vi "multiple inverters.vi"() -> ()   [LabVIEW 2018]
uses:
  <vilib>/Plasmionique/MB Master/MB_Master_TCP/MB_Master_TCP.lvclass
  <vilib>/Plasmionique/MB Master/MB Master.lvlib
  93058b94-2cfa-412c-aaea-c37432080e69.vi
  52964f07-62a9-4f69-bcdd-33621c3da344.vi
  12cb2fec-a066-4508-9dd1-fd50a70bf569.vi
  6f8febb2-9bf6-4d29-9751-6b01666fea3d.vi
  b6474e31-9fa1-4c1d-99b5-b6bb53db0f46.vi
  f1a4f3b6-1467-4be9-9e5d-893fa62d5f27.vi
  d295411a-7b3b-4ec3-9029-25cb82dd415e.vi
  31b17e4d-b534-4e5a-9b0d-c0ca24deb87e.vi
  b632eabe-c25f-4dbe-95ee-deebe4b0f4b1.vi
  7138b5ac-df4f-457e-8d99-eea4f057fb14.vi
  7631bdb0-5171-4193-ab14-fa7f9aada4b6.vi
  93641b55-29e7-4da1-9539-9e254f8d73b5.vi
  C:/Program Files (x86)/National Instruments/LabVIEW 2018/vi.lib/Plasmionique/MB Master/MB_Master/MB_Master.lvclass
panel:
  out "Curtailment  Complete":bool
  out "Power Factor Complete":bool
  out "Set Up Complete":bool
  in  "1200 Inverter IP":string
  in  "1086 Inverter IP":string
  in  "1084 Inverter IP":string
  in  "Setup Curtailment and Power Factor":bool
  in  "Send Curtailment":bool
  in  "Send Power Factor":bool
  out "Setup Runtime (s)":u16
  out "Curtailment Runtime (s)":dbl
  out "Power Factor Runtime (s)":dbl
  in  "stop":bool
  in  "Curtailment % (28-100)":enum16{""}(ring)
  in  "power Factor Setpoint":enum16{""}(ring)
  in  "Inverter Select":T1(ring)
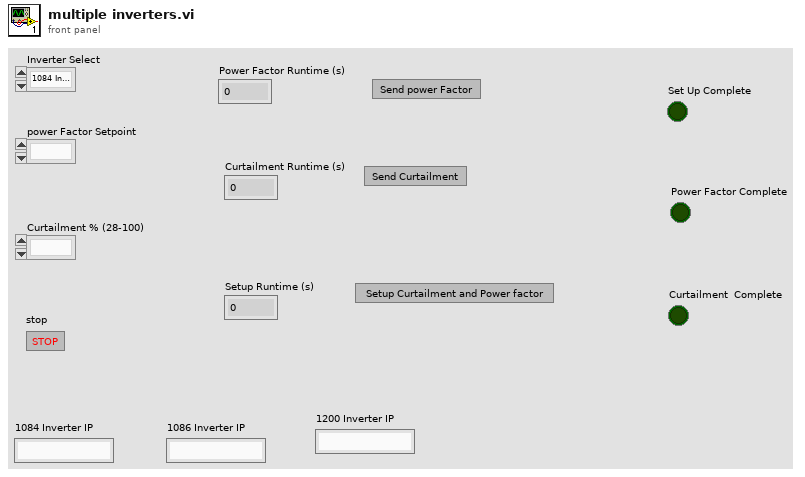
[diagram p1: front panel]
types:
  T1 = enum16{"1084 Inverter", "1086 Inverter ", "1200 Inverter"}
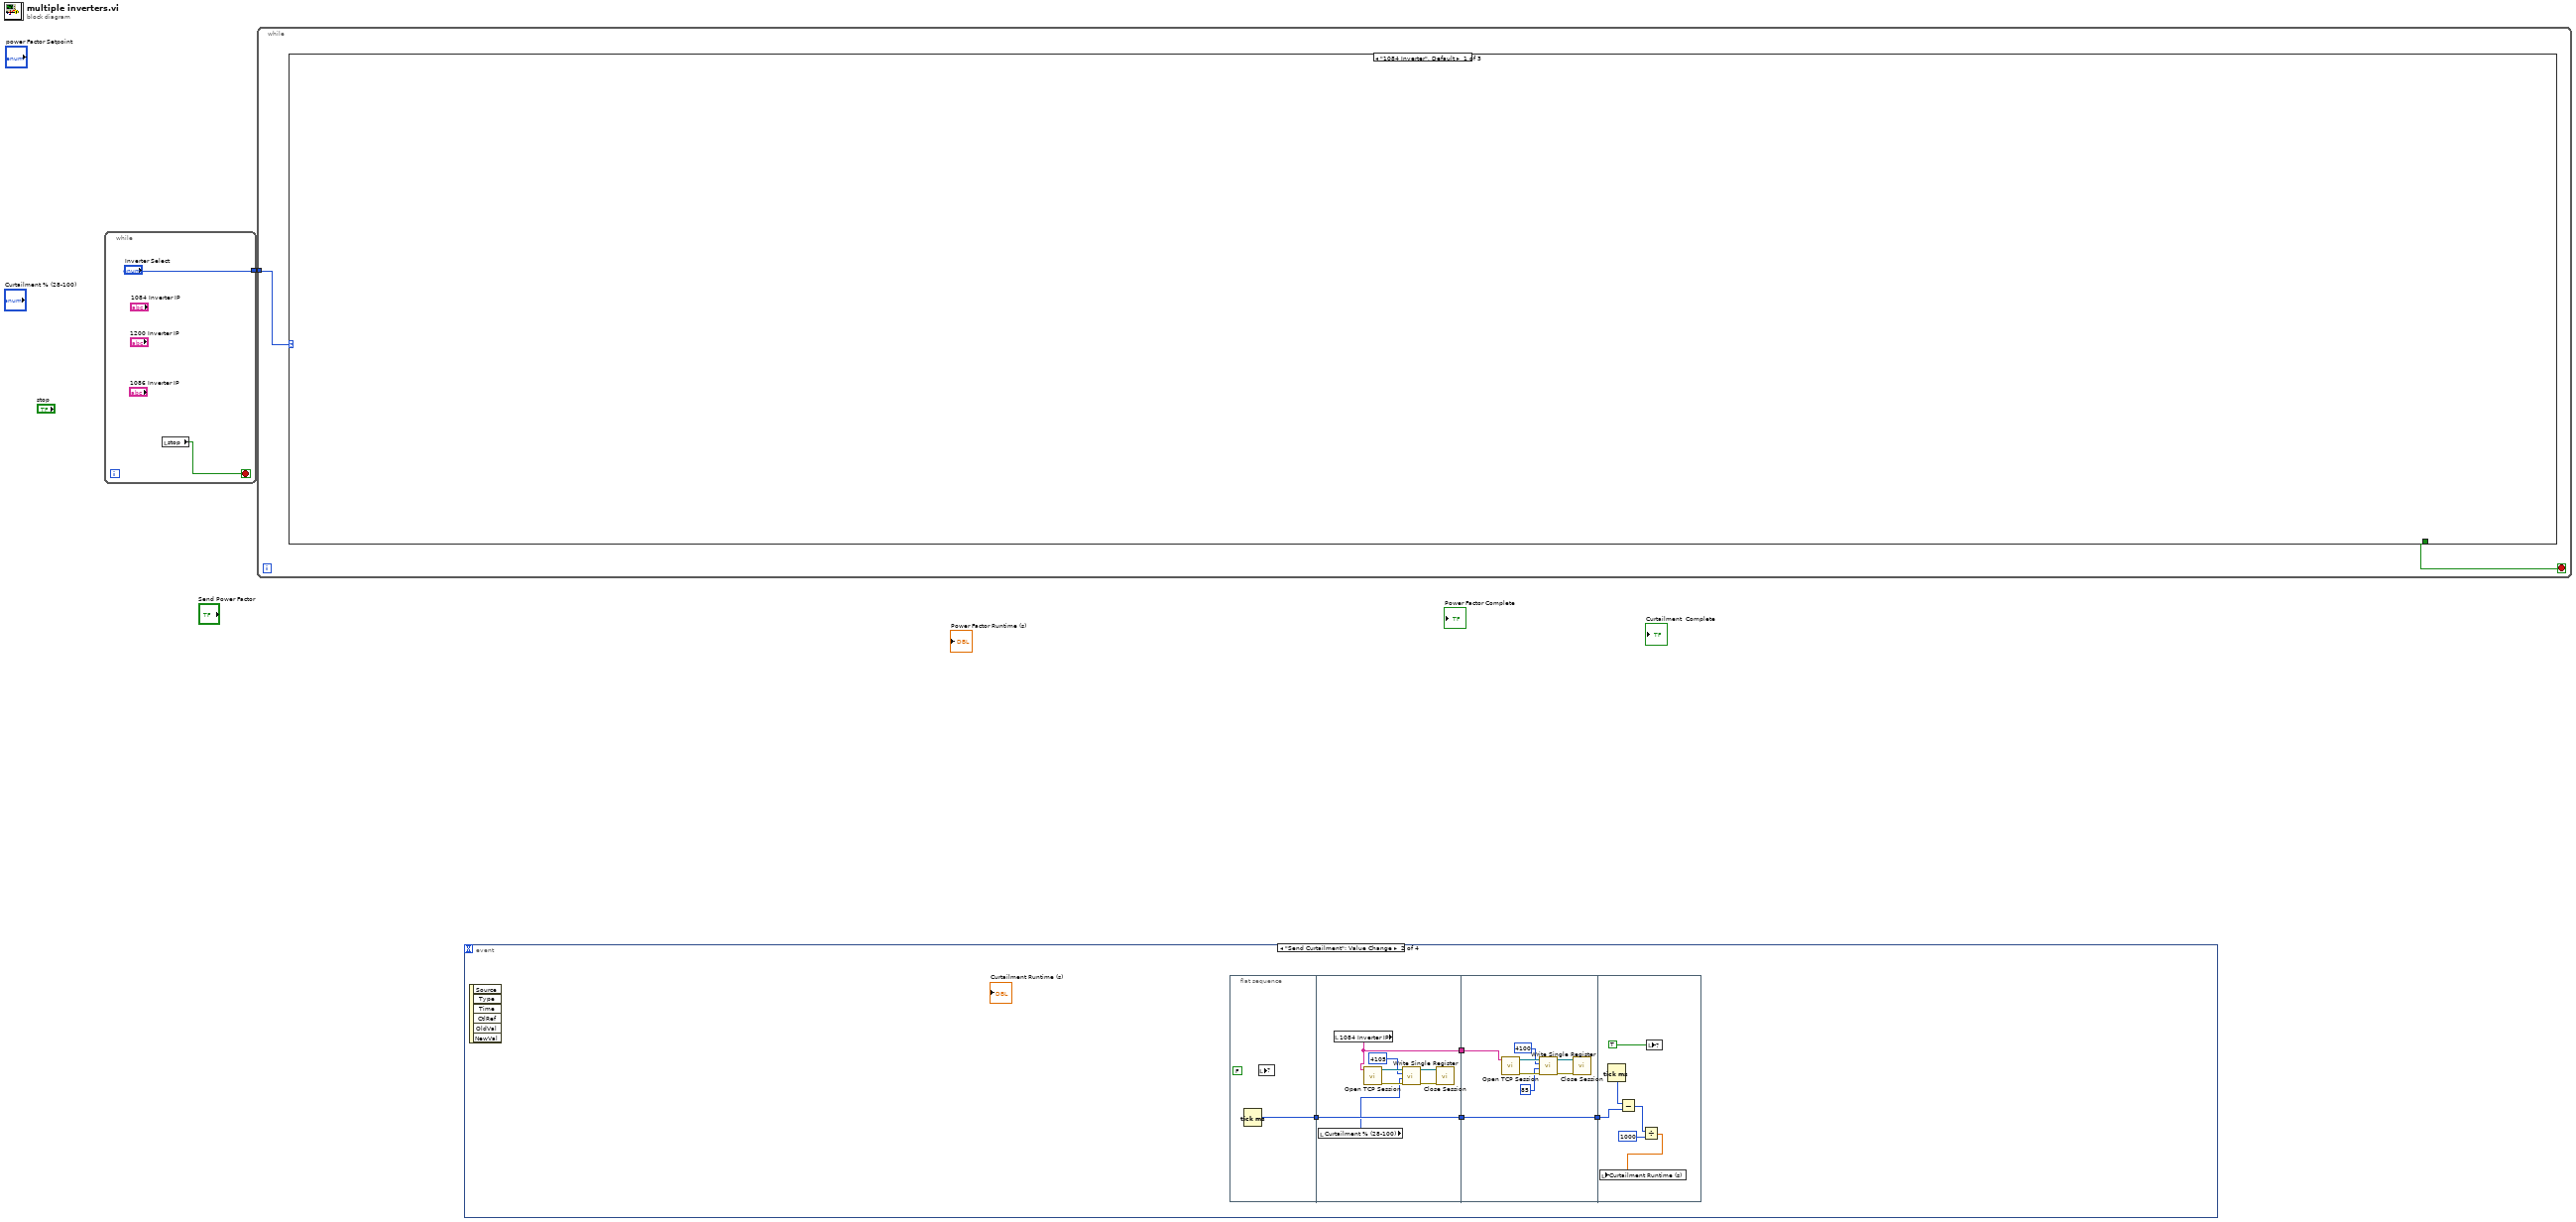
[diagram p0: block diagram]
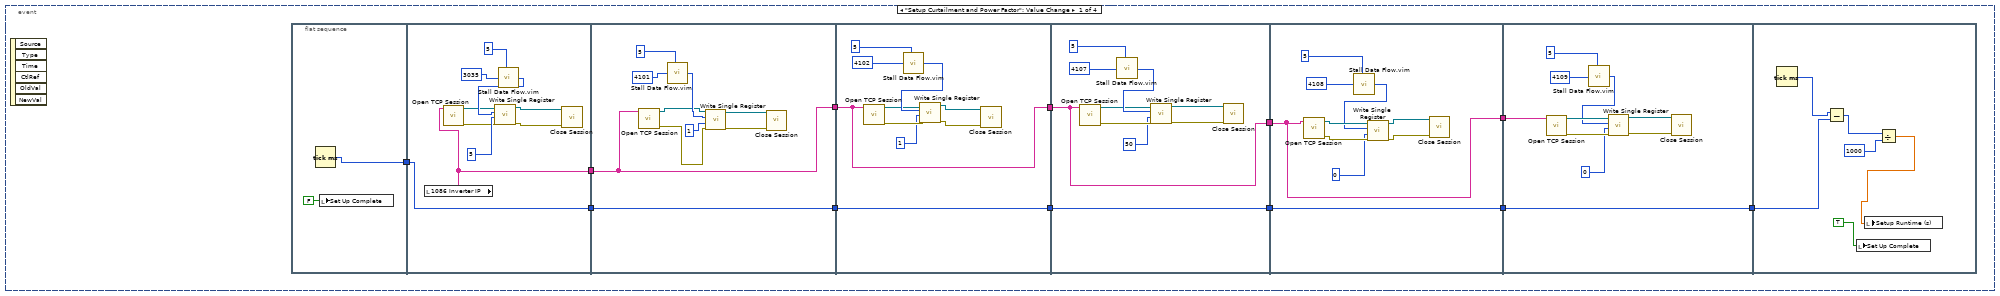
[diagram p2: hidden frame]
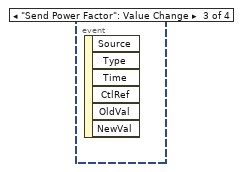
[diagram p3: hidden frame]
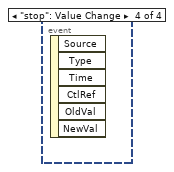
[diagram p4: hidden frame]
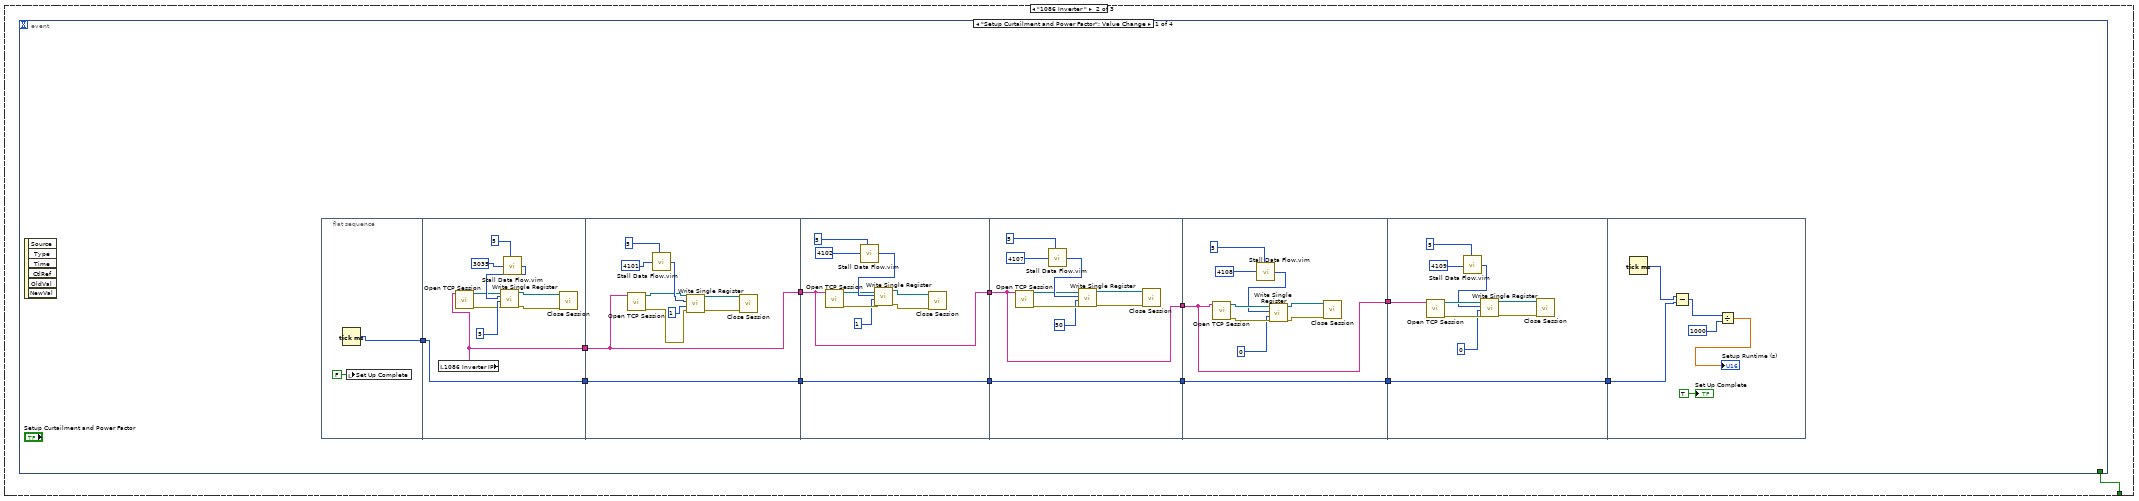
[diagram p5: hidden frame]
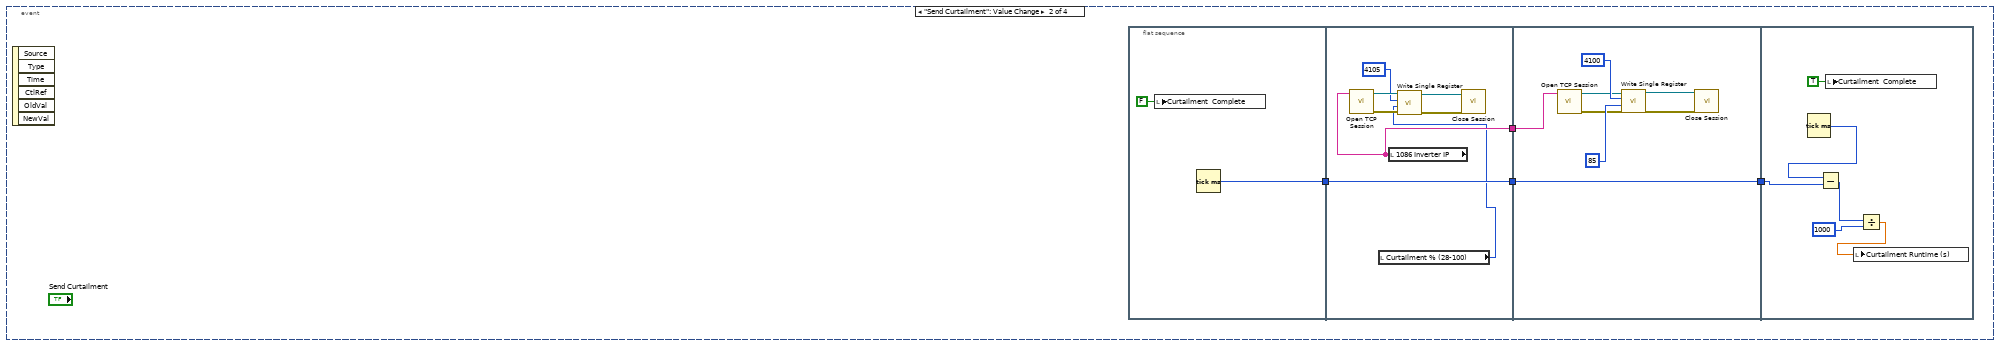
[diagram p6: hidden frame]
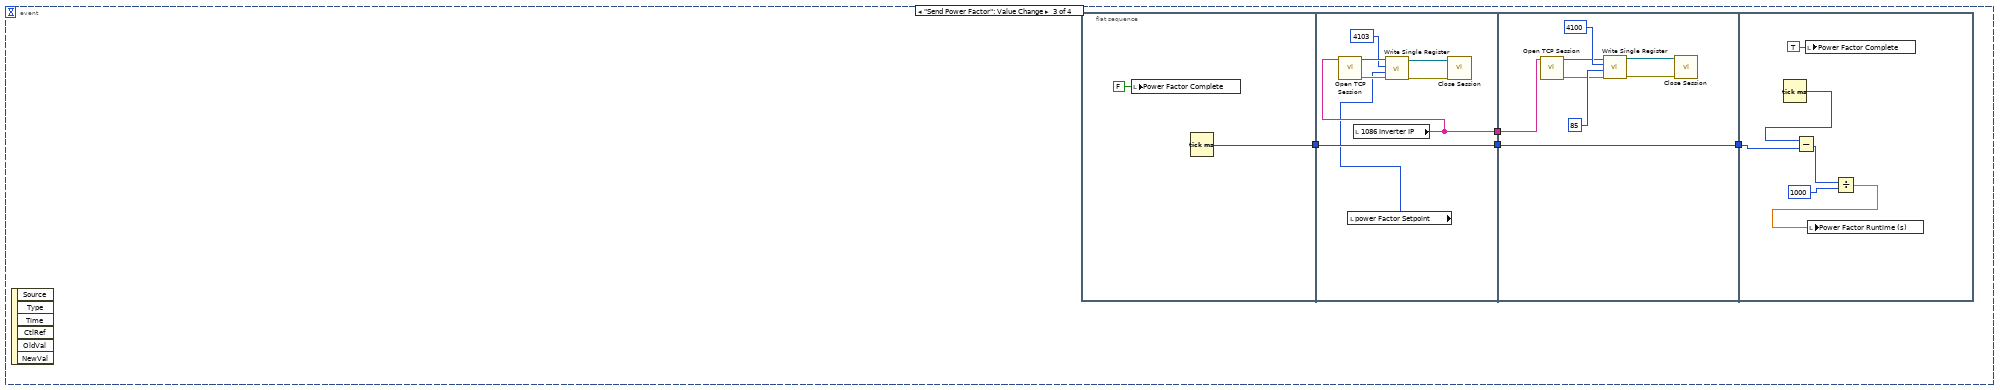
[diagram p7: hidden frame]
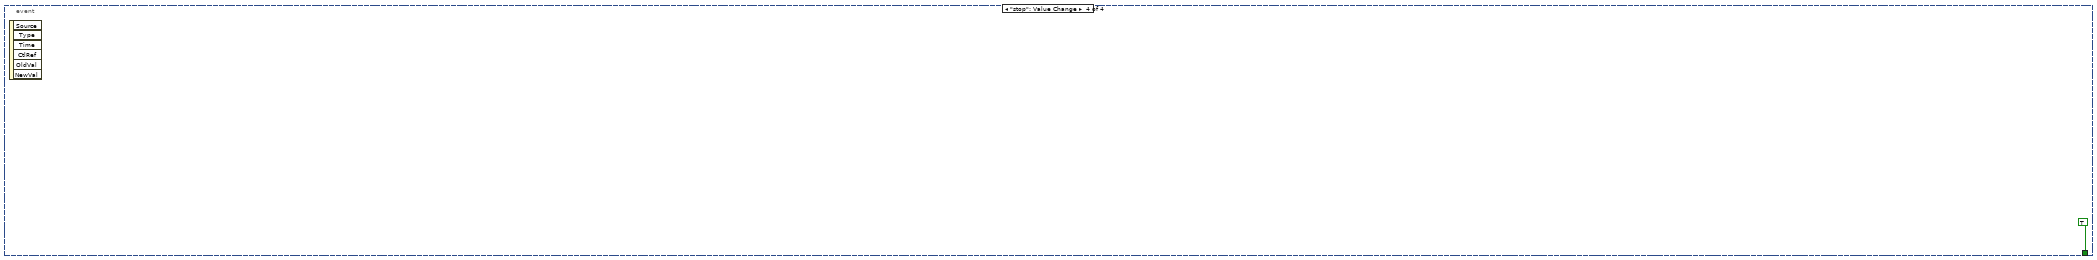
[diagram p8: hidden frame]
diagram:
  n1 = while {
    tunnel: ["Inverter Select"] -> w1
    stop <- w2 stop-if-true
    n2 = local read "stop"() -> (w2:bool)
  }
  n3 = while {
    tunnel: w1 -> [w5]
    stop <- w4 stop-if-true
    n4 = case shown="\"1084 Inverter\", Default" w5 {
      tunnel: [_ w6 _] -> w4
      frame "1084 Inverter", Default {
      }
      frame "1086 Inverter " {
        n5 = event shown="[0] \"Setup Curtailment and Power Factor\": Value Change" {
          selector: _ -> [_ _ _ _]
          dyn-events: _ -> [_ _ _ _]
          timeout: _ -> [_ _ _ _]
          tunnel: [_ _ _ TRUE] -> w6
          event "Setup Curtailment and Power Factor": Value Change {
            n6 = event-data() -> ()  [unwired: 1 in, 6 out]
            n7 = flat-sequence {
              tunnel: [w20] -> w13
              tunnel: [w22] -> w18
              tunnel: w13 -> [w21]
              tunnel: [w21] -> w12
              tunnel: w18 -> [w32]
              tunnel: [w32] -> w17
              tunnel: w12 -> [w31]
              tunnel: [w31] -> w11
              tunnel: w17 -> [w42]
              tunnel: [w42] -> w16
              tunnel: w11 -> [w41]
              tunnel: [w41] -> w10
              tunnel: w16 -> [w52]
              tunnel: [w52] -> w15
              tunnel: w10 -> [w51]
              tunnel: [w51] -> w9
              tunnel: w15 -> [w62]
              tunnel: [w62] -> w14
              tunnel: w9 -> [w61]
              tunnel: [w61] -> w8
              tunnel: w14 -> [w80]
              tunnel: w8 -> [w71]
              tunnel: [w71] -> w7
              tunnel: w7 -> [w83]
              frame #0 {
                n8 = Tick Count (ms)() -> (millisecond timer value=w20:u32)
                n9 = local write "Set Up Complete"(FALSE ("Set Up Complete")) -> ()
              }
              frame #1 {
                n10 = local read "1086 Inverter IP"() -> (w22:string)
                n11 = call <vilib>:"Open TCP Session.vi"("IP Address"=w22) -> ("error out"=w24:errorcluster, "MB_TCP session"=w26:refnum<class "MB_Master_TCP.lvclass">)  [unwired: 9 in]
                n12 = call "Stall Data Flow.vim"("value in"=3035, "milliseconds to wait"=5) -> ("value out"=w28:i32)  [unwired: 1 out]
                n13 = call <vilib>:"Write Single Register.vi"("error in (no error)"=w24, "value"=5, "address"=w28, "MB session in"=w26) -> ("error out"=w23:errorcluster, "MB session out"=w25:refnum<class "MB_Master_TCP.lvclass">)  [unwired: 6 in]
                n14 = call-dynamic "Close Session.vi"("error in (no error)"=w23, "MB TCP session"=w25) -> ()  [unwired: 9 in, 1 out]
              }
              frame #2 {
                n15 = call <vilib>:"Open TCP Session.vi"("IP Address"=w32) -> ("error out"=w34:errorcluster, "MB_TCP session"=w37:refnum<class "MB_Master_TCP.lvclass">)  [unwired: 9 in]
                n16 = call "Stall Data Flow.vim"("value in"=4101, "milliseconds to wait"=5) -> ("value out"=w38:i32)  [unwired: 1 out]
                n17 = call <vilib>:"Write Single Register.vi"("error in (no error)"=w34, "value"=1, "address"=w38, "MB session in"=w37) -> ("error out"=w33:errorcluster, "MB session out"=w36:refnum<class "MB_Master_TCP.lvclass">)  [unwired: 6 in]
                n18 = call-dynamic "Close Session.vi"("error in (no error)"=w33, "MB TCP session"=w36) -> ()  [unwired: 9 in, 1 out]
              }
              frame #3 {
                n19 = call <vilib>:"Open TCP Session.vi"("IP Address"=w42) -> ("error out"=w45:errorcluster, "MB_TCP session"=w47:refnum<class "MB_Master_TCP.lvclass">)  [unwired: 9 in]
                n20 = call "Stall Data Flow.vim"("value in"=4102, "milliseconds to wait"=5) -> ("value out"=w48:i32)  [unwired: 1 out]
                n21 = call <vilib>:"Write Single Register.vi"("error in (no error)"=w45, "value"=1, "address"=w48, "MB session in"=w47) -> ("error out"=w44:errorcluster, "MB session out"=w46:refnum<class "MB_Master_TCP.lvclass">)  [unwired: 6 in]
                n22 = call-dynamic "Close Session.vi"("error in (no error)"=w44, "MB TCP session"=w46) -> ()  [unwired: 9 in, 1 out]
              }
              frame #4 {
                n23 = call <vilib>:"Open TCP Session.vi"("IP Address"=w52) -> ("error out"=w57:errorcluster, "MB_TCP session"=w53:refnum<class "MB_Master_TCP.lvclass">)  [unwired: 9 in]
                n24 = call "Stall Data Flow.vim"("value in"=4107, "milliseconds to wait"=5) -> ("value out"=w54:i32)  [unwired: 1 out]
                n25 = call <vilib>:"Write Single Register.vi"("error in (no error)"=w57, "value"=50, "address"=w54, "MB session in"=w53) -> ("error out"=w56:errorcluster, "MB session out"=w58:refnum<class "MB_Master_TCP.lvclass">)  [unwired: 6 in]
                n26 = call-dynamic "Close Session.vi"("error in (no error)"=w56, "MB TCP session"=w58) -> ()  [unwired: 9 in, 1 out]
              }
              frame #5 {
                n27 = call <vilib>:"Open TCP Session.vi"("IP Address"=w62) -> ("error out"=w66:errorcluster, "MB_TCP session"=w68:refnum<class "MB_Master_TCP.lvclass">)  [unwired: 9 in]
                n28 = call "Stall Data Flow.vim"("value in"=4108, "milliseconds to wait"=5) -> ("value out"=w64:i32)  [unwired: 1 out]
                n29 = call <vilib>:"Write Single Register.vi"("error in (no error)"=w66, "value"=0, "address"=w64, "MB session in"=w68) -> ("error out"=w65:errorcluster, "MB session out"=w67:refnum<class "MB_Master_TCP.lvclass">)  [unwired: 6 in]
                n30 = call-dynamic "Close Session.vi"("error in (no error)"=w65, "MB TCP session"=w67) -> ()  [unwired: 9 in, 1 out]
              }
              frame #6 {
                n31 = call <vilib>:"Open TCP Session.vi"("IP Address"=w80) -> ("error out"=w77:errorcluster, "MB_TCP session"=w79:refnum<class "MB_Master_TCP.lvclass">)  [unwired: 9 in]
                n32 = call "Stall Data Flow.vim"("value in"=4109, "milliseconds to wait"=5) -> ("value out"=w73:i32)  [unwired: 1 out]
                n33 = call <vilib>:"Write Single Register.vi"("error in (no error)"=w77, "value"=0, "address"=w73, "MB session in"=w79) -> ("error out"=w76:errorcluster, "MB session out"=w78:refnum<class "MB_Master_TCP.lvclass">)  [unwired: 6 in]
                n34 = call-dynamic "Close Session.vi"("error in (no error)"=w76, "MB TCP session"=w78) -> ()  [unwired: 9 in, 1 out]
              }
              frame #7 {
                n35 = Tick Count (ms)() -> (millisecond timer value=w84:u32)
                n36 = Subtract(x=w84, y=w83) -> (x-y=w86:u32)
                n37 = Divide(x=w86, y=1000) -> (x/y=→"Setup Runtime (s)":dbl)
                "Set Up Complete" <- TRUE ("Set Up Complete")
              }
            }
          }
          event "Send Curtailment": Value Change {
            n38 = event-data() -> ()  [unwired: 1 in, 6 out]
            n39 = flat-sequence {
              tunnel: [w92] -> w90
              tunnel: w90 -> [w100]
              tunnel: [w100] -> w89
              tunnel: [w94] -> w87
              tunnel: w89 -> [w108]
              tunnel: [w108] -> w88
              tunnel: w87 -> [w101]
              tunnel: w88 -> [w113]
              frame #0 {
                n40 = local write "Curtailment  Complete"(FALSE ("Curtailment  Complete")) -> ()
                n41 = Tick Count (ms)() -> (millisecond timer value=w92:u32)
              }
              frame #1 {
                n42 = local read "Curtailment % (28-100)"() -> (w93:enum16{""})
                n43 = local read "1086 Inverter IP"() -> (w94:string)
                n44 = call <vilib>:"Open TCP Session.vi"("IP Address"=w94) -> ("error out"=w97:errorcluster, "MB_TCP session"=w99:refnum<class "MB_Master_TCP.lvclass">)  [unwired: 9 in]
                n45 = call <vilib>:"Write Single Register.vi"("error in (no error)"=w97, "value"=w93, "address"=4105, "MB session in"=w99) -> ("error out"=w96:errorcluster, "MB session out"=w98:refnum<class "MB_Master_TCP.lvclass">)  [unwired: 6 in]
                n46 = call-dynamic "Close Session.vi"("error in (no error)"=w96, "MB TCP session"=w98) -> ()  [unwired: 9 in, 1 out]
              }
              frame #2 {
                n47 = call <vilib>:"Open TCP Session.vi"("IP Address"=w101) -> ("error out"=w103:errorcluster, "MB_TCP session"=w105:refnum<class "MB_Master_TCP.lvclass">)  [unwired: 9 in]
                n48 = call <vilib>:"Write Single Register.vi"("error in (no error)"=w103, "value"=85, "address"=4100, "MB session in"=w105) -> ("error out"=w102:errorcluster, "MB session out"=w104:refnum<class "MB_Master_TCP.lvclass">)  [unwired: 6 in]
                n49 = call-dynamic "Close Session.vi"("error in (no error)"=w102, "MB TCP session"=w104) -> ()  [unwired: 9 in, 1 out]
              }
              frame #3 {
                n50 = Tick Count (ms)() -> (millisecond timer value=w114:u32)
                n51 = Subtract(x=w114, y=w113) -> (x-y=w112:u32)
                n52 = local write "Curtailment  Complete"(TRUE ("Curtailment  Complete")) -> ()
                n53 = Divide(x=w112, y=1000) -> (x/y=w110:dbl)
                n54 = local write "Curtailment Runtime (s)"(w110) -> ()
              }
            }
          }
          event "Send Power Factor": Value Change {
            n55 = event-data() -> ()  [unwired: 1 in, 6 out]
            n56 = flat-sequence {
              tunnel: [w120] -> w118
              tunnel: w118 -> [w128]
              tunnel: [w128] -> w117
              tunnel: [w122] -> w115
              tunnel: w117 -> [w136]
              tunnel: [w136] -> w116
              tunnel: w115 -> [w129]
              tunnel: w116 -> [w141]
              frame #0 {
                n57 = local write "Power Factor Complete"(FALSE ("Power Factor Complete")) -> ()
                n58 = Tick Count (ms)() -> (millisecond timer value=w120:u32)
              }
              frame #1 {
                n59 = local read "power Factor Setpoint"() -> (w121:enum16{""})
                n60 = local read "1086 Inverter IP"() -> (w122:string)
                n61 = call <vilib>:"Open TCP Session.vi"("IP Address"=w122) -> ("error out"=w125:errorcluster, "MB_TCP session"=w127:refnum<class "MB_Master_TCP.lvclass">)  [unwired: 9 in]
                n62 = call <vilib>:"Write Single Register.vi"("error in (no error)"=w125, "value"=w121, "address"=4103, "MB session in"=w127) -> ("error out"=w124:errorcluster, "MB session out"=w126:refnum<class "MB_Master_TCP.lvclass">)  [unwired: 6 in]
                n63 = call-dynamic "Close Session.vi"("error in (no error)"=w124, "MB TCP session"=w126) -> ()  [unwired: 9 in, 1 out]
              }
              frame #2 {
                n64 = call <vilib>:"Open TCP Session.vi"("IP Address"=w129) -> ("error out"=w131:errorcluster, "MB_TCP session"=w133:refnum<class "MB_Master_TCP.lvclass">)  [unwired: 9 in]
                n65 = call <vilib>:"Write Single Register.vi"("error in (no error)"=w131, "value"=85, "address"=4100, "MB session in"=w133) -> ("error out"=w130:errorcluster, "MB session out"=w132:refnum<class "MB_Master_TCP.lvclass">)  [unwired: 6 in]
                n66 = call-dynamic "Close Session.vi"("error in (no error)"=w130, "MB TCP session"=w132) -> ()  [unwired: 9 in, 1 out]
              }
              frame #3 {
                n67 = Tick Count (ms)() -> (millisecond timer value=w142:u32)
                n68 = Subtract(x=w142, y=w141) -> (x-y=w140:u32)
                n69 = local write "Power Factor Complete"(TRUE ("Power Factor Complete")) -> ()
                n70 = Divide(x=w140, y=1000) -> (x/y=w137:dbl)
                n71 = local write "Power Factor Runtime (s)"(w137) -> ()
              }
            }
          }
          event "stop": Value Change {
            n72 = event-data() -> ()  [unwired: 1 in, 6 out]
          }
        }
      }
      frame "1200 Inverter" {
      }
    }
  }
  n73 = event shown="[1] \"Send Curtailment\": Value Change" {
    selector: _ -> [_ _ _ _]
    dyn-events: _ -> [_ _ _ _]
    timeout: _ -> [_ _ _ _]
    event "Setup Curtailment and Power Factor": Value Change {
      n74 = event-data() -> ()  [unwired: 1 in, 6 out]
      n75 = flat-sequence {
        tunnel: [w157] -> w155
        tunnel: [w159] -> w154
        tunnel: w155 -> [w158]
        tunnel: [w158] -> w153
        tunnel: w154 -> [w169]
        tunnel: [w169] -> w152
        tunnel: w153 -> [w168]
        tunnel: [w168] -> w151
        tunnel: w152 -> [w179]
        tunnel: [w179] -> w150
        tunnel: w151 -> [w178]
        tunnel: [w178] -> w149
        tunnel: w150 -> [w189]
        tunnel: [w189] -> w148
        tunnel: w149 -> [w188]
        tunnel: [w188] -> w147
        tunnel: w148 -> [w199]
        tunnel: [w199] -> w146
        tunnel: w147 -> [w198]
        tunnel: [w198] -> w145
        tunnel: w146 -> [w217]
        tunnel: w145 -> [w208]
        tunnel: [w208] -> w144
        tunnel: w144 -> [w220]
        frame #0 {
          n76 = Tick Count (ms)() -> (millisecond timer value=w157:u32)
          n77 = local write "Set Up Complete"(FALSE ("Set Up Complete")) -> ()
        }
        frame #1 {
          n78 = local read "1086 Inverter IP"() -> (w159:string)
          n79 = call <vilib>:"Open TCP Session.vi"("IP Address"=w159) -> ("error out"=w161:errorcluster, "MB_TCP session"=w163:refnum<class "MB_Master_TCP.lvclass">)  [unwired: 9 in]
          n80 = call "Stall Data Flow.vim"("value in"=3035, "milliseconds to wait"=5) -> ("value out"=w165:i32)  [unwired: 1 out]
          n81 = call <vilib>:"Write Single Register.vi"("error in (no error)"=w161, "value"=5, "address"=w165, "MB session in"=w163) -> ("error out"=w160:errorcluster, "MB session out"=w162:refnum<class "MB_Master_TCP.lvclass">)  [unwired: 6 in]
          n82 = call-dynamic "Close Session.vi"("error in (no error)"=w160, "MB TCP session"=w162) -> ()  [unwired: 9 in, 1 out]
        }
        frame #2 {
          n83 = call <vilib>:"Open TCP Session.vi"("IP Address"=w169) -> ("error out"=w171:errorcluster, "MB_TCP session"=w174:refnum<class "MB_Master_TCP.lvclass">)  [unwired: 9 in]
          n84 = call "Stall Data Flow.vim"("value in"=4101, "milliseconds to wait"=5) -> ("value out"=w175:i32)  [unwired: 1 out]
          n85 = call <vilib>:"Write Single Register.vi"("error in (no error)"=w171, "value"=1, "address"=w175, "MB session in"=w174) -> ("error out"=w170:errorcluster, "MB session out"=w173:refnum<class "MB_Master_TCP.lvclass">)  [unwired: 6 in]
          n86 = call-dynamic "Close Session.vi"("error in (no error)"=w170, "MB TCP session"=w173) -> ()  [unwired: 9 in, 1 out]
        }
        frame #3 {
          n87 = call <vilib>:"Open TCP Session.vi"("IP Address"=w179) -> ("error out"=w182:errorcluster, "MB_TCP session"=w184:refnum<class "MB_Master_TCP.lvclass">)  [unwired: 9 in]
          n88 = call "Stall Data Flow.vim"("value in"=4102, "milliseconds to wait"=5) -> ("value out"=w185:i32)  [unwired: 1 out]
          n89 = call <vilib>:"Write Single Register.vi"("error in (no error)"=w182, "value"=1, "address"=w185, "MB session in"=w184) -> ("error out"=w181:errorcluster, "MB session out"=w183:refnum<class "MB_Master_TCP.lvclass">)  [unwired: 6 in]
          n90 = call-dynamic "Close Session.vi"("error in (no error)"=w181, "MB TCP session"=w183) -> ()  [unwired: 9 in, 1 out]
        }
        frame #4 {
          n91 = call <vilib>:"Open TCP Session.vi"("IP Address"=w189) -> ("error out"=w194:errorcluster, "MB_TCP session"=w190:refnum<class "MB_Master_TCP.lvclass">)  [unwired: 9 in]
          n92 = call "Stall Data Flow.vim"("value in"=4107, "milliseconds to wait"=5) -> ("value out"=w191:i32)  [unwired: 1 out]
          n93 = call <vilib>:"Write Single Register.vi"("error in (no error)"=w194, "value"=50, "address"=w191, "MB session in"=w190) -> ("error out"=w193:errorcluster, "MB session out"=w195:refnum<class "MB_Master_TCP.lvclass">)  [unwired: 6 in]
          n94 = call-dynamic "Close Session.vi"("error in (no error)"=w193, "MB TCP session"=w195) -> ()  [unwired: 9 in, 1 out]
        }
        frame #5 {
          n95 = call <vilib>:"Open TCP Session.vi"("IP Address"=w199) -> ("error out"=w203:errorcluster, "MB_TCP session"=w205:refnum<class "MB_Master_TCP.lvclass">)  [unwired: 9 in]
          n96 = call "Stall Data Flow.vim"("value in"=4108, "milliseconds to wait"=5) -> ("value out"=w201:i32)  [unwired: 1 out]
          n97 = call <vilib>:"Write Single Register.vi"("error in (no error)"=w203, "value"=0, "address"=w201, "MB session in"=w205) -> ("error out"=w202:errorcluster, "MB session out"=w204:refnum<class "MB_Master_TCP.lvclass">)  [unwired: 6 in]
          n98 = call-dynamic "Close Session.vi"("error in (no error)"=w202, "MB TCP session"=w204) -> ()  [unwired: 9 in, 1 out]
        }
        frame #6 {
          n99 = call <vilib>:"Open TCP Session.vi"("IP Address"=w217) -> ("error out"=w214:errorcluster, "MB_TCP session"=w216:refnum<class "MB_Master_TCP.lvclass">)  [unwired: 9 in]
          n100 = call "Stall Data Flow.vim"("value in"=4109, "milliseconds to wait"=5) -> ("value out"=w210:i32)  [unwired: 1 out]
          n101 = call <vilib>:"Write Single Register.vi"("error in (no error)"=w214, "value"=0, "address"=w210, "MB session in"=w216) -> ("error out"=w213:errorcluster, "MB session out"=w215:refnum<class "MB_Master_TCP.lvclass">)  [unwired: 6 in]
          n102 = call-dynamic "Close Session.vi"("error in (no error)"=w213, "MB TCP session"=w215) -> ()  [unwired: 9 in, 1 out]
        }
        frame #7 {
          n103 = Tick Count (ms)() -> (millisecond timer value=w221:u32)
          n104 = Subtract(x=w221, y=w220) -> (x-y=w223:u32)
          n105 = local write "Set Up Complete"(TRUE ("Set Up Complete")) -> ()
          n106 = Divide(x=w223, y=1000) -> (x/y=w218:dbl)
          n107 = local write "Setup Runtime (s)"(w218) -> ()
        }
      }
    }
    event "Send Curtailment": Value Change {
      n108 = event-data() -> ()  [unwired: 1 in, 6 out]
      n109 = flat-sequence {
        tunnel: [w228] -> w227
        tunnel: w227 -> [w231]
        tunnel: [w231] -> w226
        tunnel: [w230] -> w225
        tunnel: [w244] -> w224
        tunnel: w226 -> [w244]
        tunnel: w225 -> [w237]
        tunnel: w224 -> [w249]
        frame #0 {
          (unwired) FALSE ("Curtailment Sent")
          n110 = Tick Count (ms)() -> (millisecond timer value=w228:u32)
          n111 = local read item#-1() -> ()  [unwired: 1 in]
        }
        frame #1 {
          n112 = local read "Curtailment % (28-100)"() -> (w229:enum16{""})
          n113 = local read "1084 Inverter IP"() -> (w230:string)
          n114 = call <vilib>:"Open TCP Session.vi"("IP Address"=w230) -> ("error out"=w234:errorcluster, "MB_TCP session"=w236:refnum<class "MB_Master_TCP.lvclass">)  [unwired: 9 in]
          n115 = call <vilib>:"Write Single Register.vi"("error in (no error)"=w234, "value"=w229, "address"=u16 4105, "MB session in"=w236) -> ("error out"=w233:errorcluster, "MB session out"=w232:refnum<class "MB_Master_TCP.lvclass">)  [unwired: 6 in]
          n116 = call-dynamic "Close Session.vi"("error in (no error)"=w233, "MB TCP session"=w232) -> ()  [unwired: 9 in, 1 out]
        }
        frame #2 {
          n117 = call <vilib>:"Open TCP Session.vi"("IP Address"=w237) -> ("error out"=w241:errorcluster, "MB_TCP session"=w243:refnum<class "MB_Master_TCP.lvclass">)  [unwired: 9 in]
          n118 = call <vilib>:"Write Single Register.vi"("error in (no error)"=w241, "value"=u16 85, "address"=u16 4100, "MB session in"=w243) -> ("error out"=w240:errorcluster, "MB session out"=w239:refnum<class "MB_Master_TCP.lvclass">)  [unwired: 6 in]
          n119 = call-dynamic "Close Session.vi"("error in (no error)"=w240, "MB TCP session"=w239) -> ()  [unwired: 9 in, 1 out]
        }
        frame #3 {
          n120 = Tick Count (ms)() -> (millisecond timer value=w250:u32)
          n121 = Subtract(x=w250, y=w249) -> (x-y=w248:u32)
          n122 = Divide(x=w248, y=u32 1000) -> (x/y=w245:dbl)
          n123 = local write "Curtailment Runtime (s)"(w245) -> ()
          n124 = local write item#-1(TRUE ("Curtailment Sent")) -> ()
        }
      }
    }
    event "Send Power Factor": Value Change {
      n125 = event-data() -> ()  [unwired: 1 in, 6 out]
    }
    event "stop": Value Change {
      n126 = event-data() -> ()  [unwired: 1 in, 6 out]
    }
  }
